vi "AccelnetPIDCtrl.vi"(6 "Control Mode":T3, 7 "Gen Control":T1, 8 "Motor actual velocity (rad/s)":dbl, 9 "Velocity setpoint (rad/s)":dbl, 10 "Torque Sensor (Nm)":dbl, 11 "Torque Setpoint (Nm)":dbl) -> (3 "Torque demand (Nm)":dbl)   [LabVIEW 2018]
uses:
  Clusters/GenCtrlMode.ctl
  Clusters/GenCtrl.ctl
  Clusters/GenMode.ctl
  <vilib>/ptbypt/NI_PtbyPt.lvlib
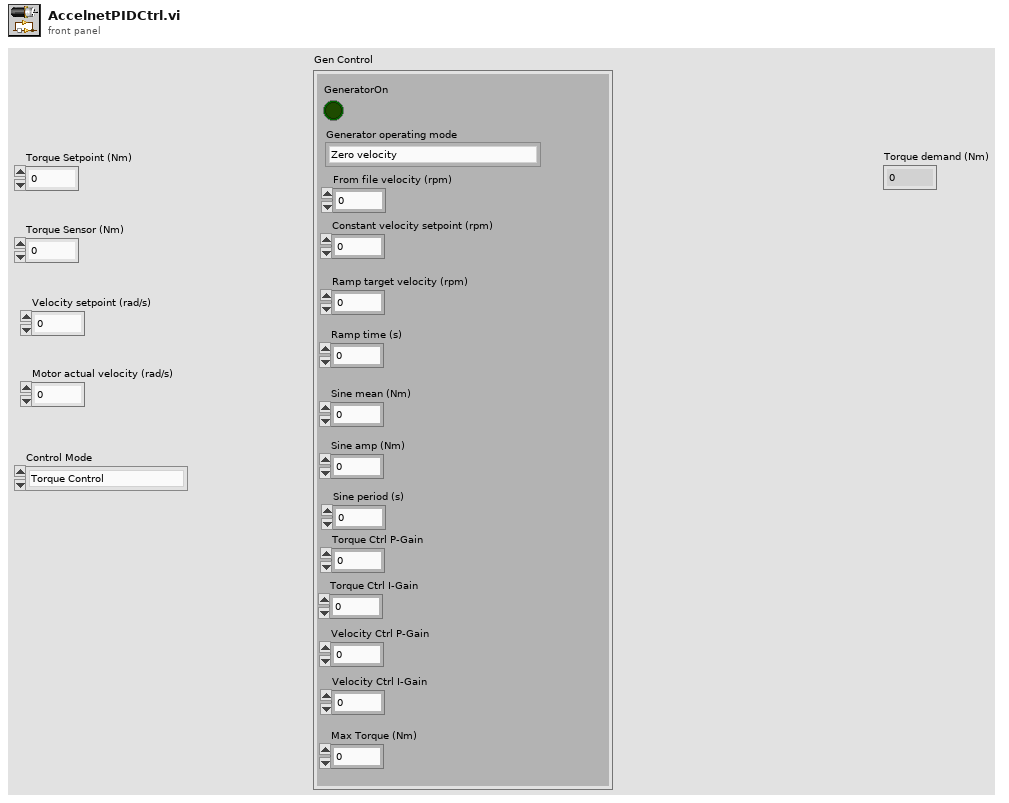
[diagram p1: front panel]
types:
  T1 = typedef "GenCtrl.ctl" = cluster{"Generator operating mode":T2, "Constant velocity setpoint (rpm)":dbl, "Ramp target velocity (rpm)":dbl, "Ramp time (s)":dbl, "Sine mean (Nm)":dbl, "Sine amp (Nm)":dbl, "Sine period (s)":dbl, "Torque Ctrl I-Gain":dbl, "Velocity Ctrl P-Gain":dbl, "Velocity Ctrl I-Gain":dbl, "Max Torque (Nm)":dbl, "GeneratorOn":bool, "Torque Ctrl P-Gain":dbl, "From file velocity (rpm)":dbl}
  T2 = typedef "GenMode.ctl" = enum16{"Zero velocity", "Velocity from File", "Constant velocity", "Ramped Velocity", "Sine Torque", "ROSCO"}
  T3 = typedef "GenCtrlMode.ctl" = enum16{"Torque Control", "Velocity Control"}
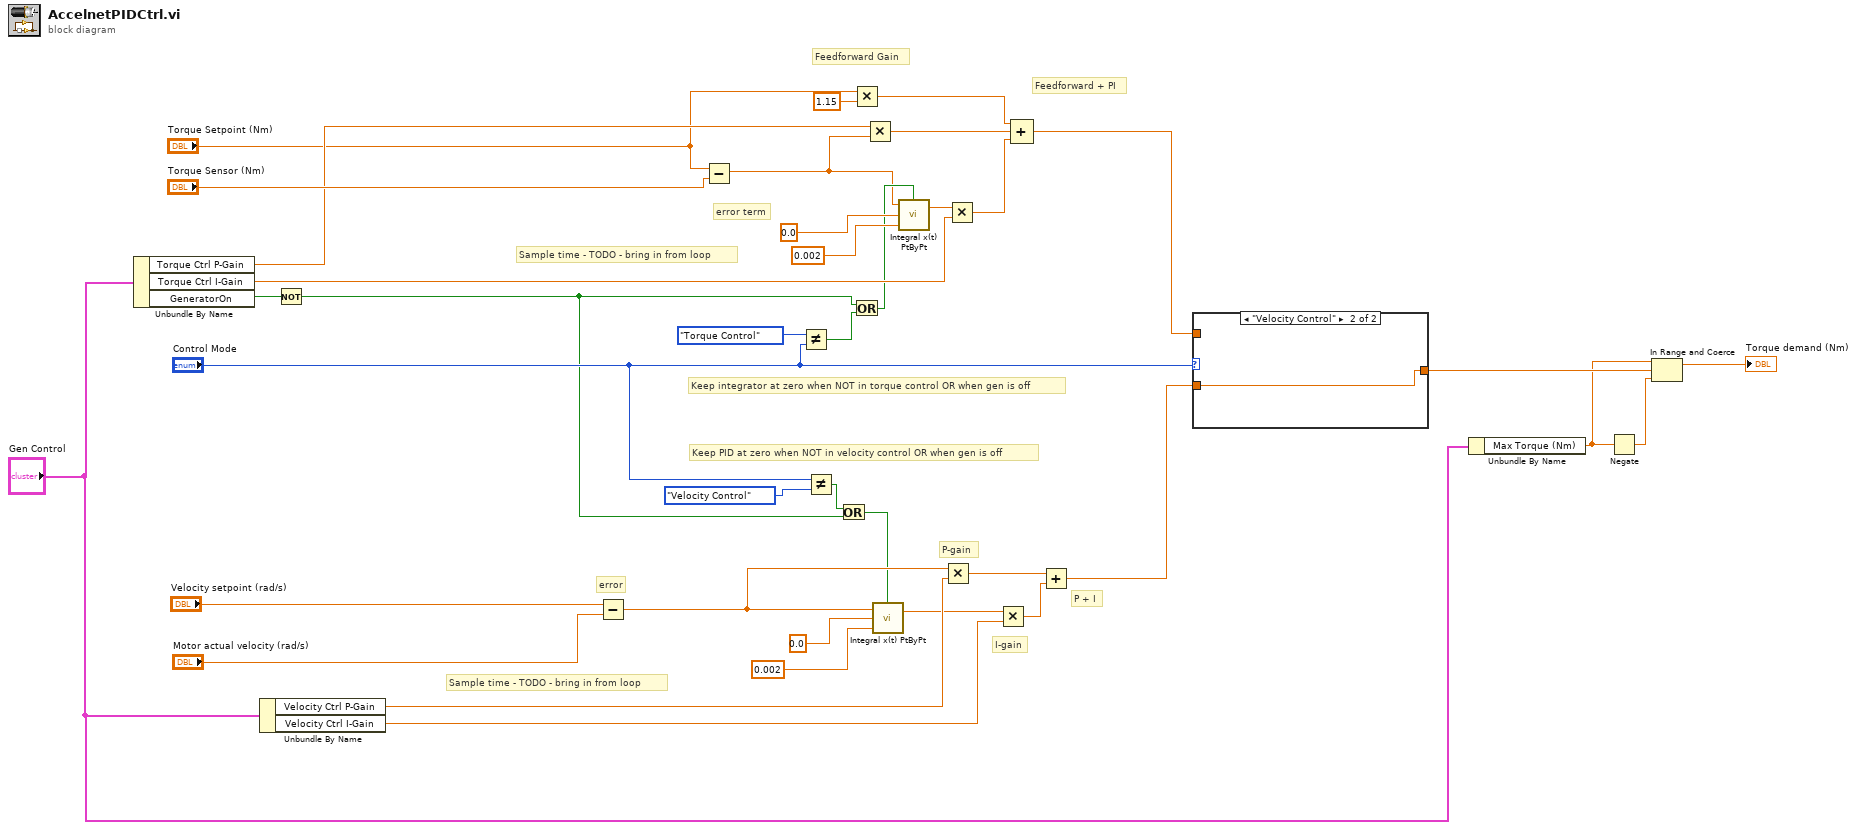
[diagram p0: block diagram]
diagram:
  # "Feedforward Gain"
  # "Sample time - TODO - bring in from loop"
  # "error"
  # "P + I"
  # "I-gain"
  # "P-gain"
  # "Keep PID at zero when NOT in velocity control OR when gen is off"
  # "Keep integrator at zero when NOT in torque control OR when gen is off"
  # "Sample time - TODO - bring in from loop"
  # "error term"
  # "Feedforward + PI"
  n1 = Unbundle By Name("Gen Control") -> ("Torque Ctrl P-Gain"=w4:dbl, "Torque Ctrl I-Gain"=w31:dbl, "GeneratorOn"=w15:bool)
  n2 = Unbundle By Name("Gen Control") -> ("Velocity Ctrl P-Gain"=w25:dbl, "Velocity Ctrl I-Gain"=w23:dbl)
  n3 = Not(x=w15) -> (.not. x?=w11:bool)
  n4 = Subtract(x="Velocity setpoint (rad/s)", y="Motor actual velocity (rad/s)") -> (x-y=w26:dbl)
  n5 = Subtract(x="Torque Setpoint (Nm)", y="Torque Sensor (Nm)") -> (x-y=w8:dbl)
  n6 = Not Equal?(x=GenCtrlMode."Torque Control" ("Control Mode"), y="Control Mode") -> (x != y?=w14:bool)
  n7 = Not Equal?(x="Control Mode", y=GenCtrlMode."Velocity Control" ("Control Mode")) -> (x != y?=w12:bool)
  n8 = Or(x=w12, y=w11) -> (x .or. y?=w10:bool)
  n9 = Multiply(x="Torque Setpoint (Nm)", y=1.15) -> (x*y=w1:dbl)
  n10 = Or(x=w11, y=w14) -> (x .or. y?=w13:bool)
  n11 = Multiply(x=w4, y=w8) -> (x*y=w6:dbl)
  n12 = call <vilib>:"Integral x(t) PtByPt.vi"("initialize"=w10, "dt"=0.002 ("dt (s)"), "initial condition"=0.0, "x"=w26) -> ("integral x(t)"=w24:dbl)  [unwired: 1 out]
  n13 = call <vilib>:"Integral x(t) PtByPt.vi"("initialize"=w13, "dt"=0.002, "initial condition"=0.0, "x"=w8) -> ("integral x(t)"=w36:dbl)  [unwired: 1 out]
  n14 = Multiply(x=w26, y=w25) -> (x*y=w9:dbl)
  n15 = Multiply(x=w36, y=w31) -> (x*y=w5:dbl)
  n16 = Multiply(x=w24, y=w23) -> (x*y=w22:dbl)
  n17 = Compound Arithmetic op=ADD(w1, w6, w5) -> (w7:dbl)
  n18 = Add(x=w9, y=w22) -> (x+y=w21:dbl)
  n19 = case shown="\"Velocity Control\"" "Control Mode" {
    tunnel: w7 -> [w39 _]
    tunnel: [w39 w40] -> w19
    tunnel: w21 -> [_ w40]
    frame "Torque Control", Default {
    }
    frame "Velocity Control" {
    }
  }
  n20 = Unbundle By Name("Gen Control") -> ("Max Torque (Nm)"=w18:dbl)
  n21 = Negate(x=w18) -> (-x=w17:dbl)
  n22 = In Range and Coerce(upper limit=w18, x=w19, lower limit=w17) -> (coerced(x)=→"Torque demand (Nm)":dbl)  [unwired: 1 out]
